vi "PDF Optionen automatisch.vi"(8 "error in (no error)":errorcluster caption="Fehler (Eingang, kein Fehler)", 9 "PDF Optionen Referenzen Cluster":T1, 10 "Anzahl aktive Komponenten":i32, 11 "PDF Optionen (Eingang)":T2) -> (0 "error out":errorcluster caption="Fehler (Ausgang)", 2 "Anzahl aktive Komponenten out":i32, 3 "PDF Optionen (Ausgang)":T2, 4 "PDF Einzelseiten Span":bool, 5 "PDF öffnen":bool, 6 "PDF Einzelseiten Komponenten":bool, 7 "PDF Deckblatt":bool)   [LabVIEW 2020, in "Linearisierung v2.lvlib" / "Protokoll.lvlib"]
uses:
  Protokoll.lvlib
  SpanEinstellungen/PDF Optionen.ctl
  SpanEinstellungen/SpanEinstellungen.lvlib
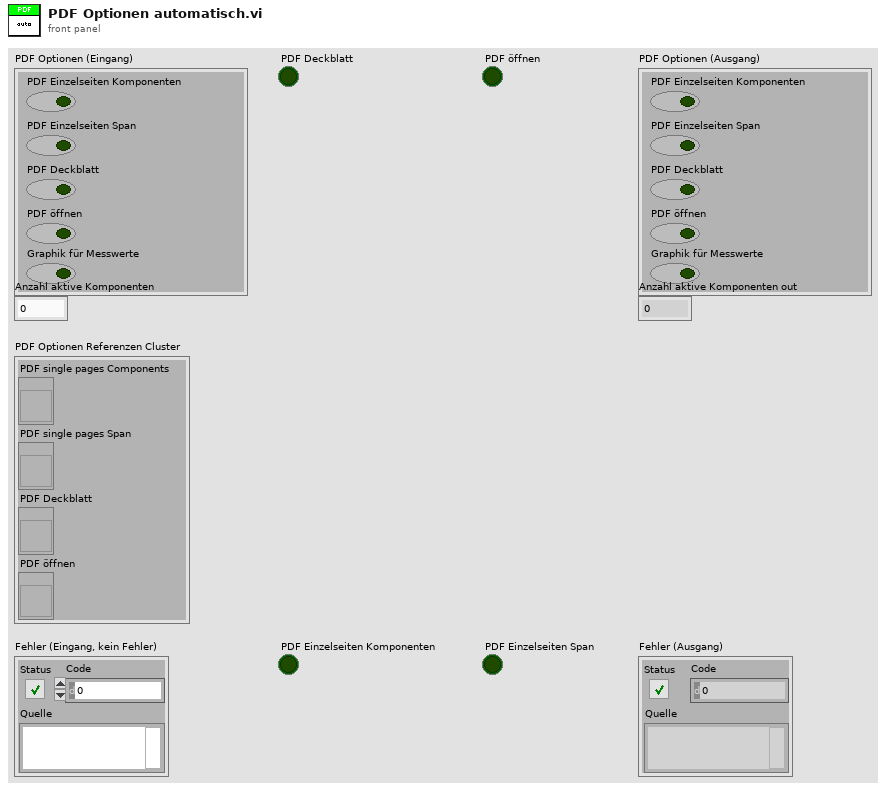
[diagram p1: front panel]
types:
  T1 = cluster{"PDF single pages Components":refnum<vi>, "PDF single pages Span":refnum<vi>, "PDF Deckblatt":refnum<vi>, "PDF öffnen":refnum<vi>}
  T2 = typedef "Linearisierung v2.lvlib/SpanEinstellungen.lvlib/PDF Optionen.ctl" = cluster{"PDF Einzelseiten Komponenten":bool, "PDF Einzelseiten Span":bool, "PDF Deckblatt":bool, "PDF öffnen":bool, "Graphik für Messwerte":bool}
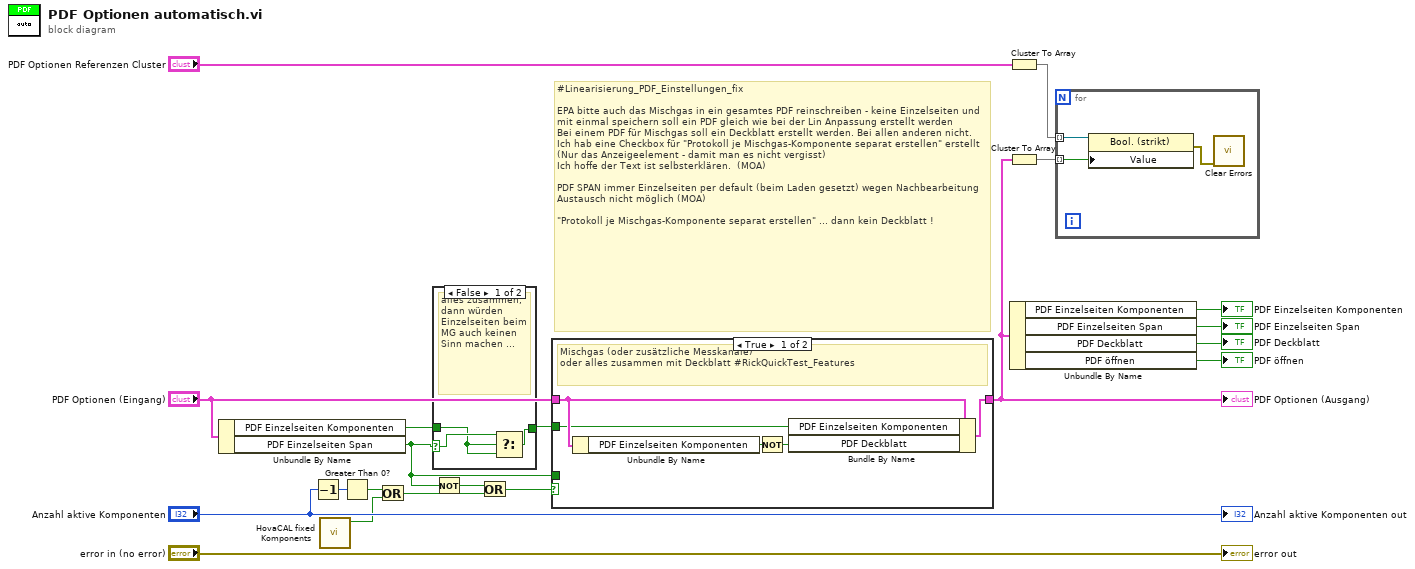
[diagram p0: block diagram]
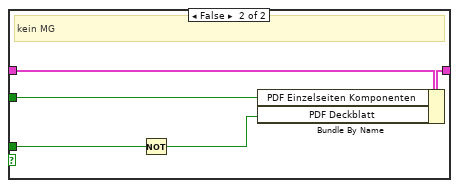
[diagram p3: hidden frame]
diagram:
  # "#Linearisierung_PDF_Einstellungen_fix\n\nEPA bitte auch das Mischgas in ein gesamtes PDF reinschreiben - keine Einzelseiten und mit einmal speichern soll ein PDF gleich wie bei der Lin Anpassung erstellt werden\nBei einem PDF für Mischgas soll ein Deckblatt erstellt werden. Bei allen anderen nicht. \nIch hab eine Checkbox für \"Protokoll je Mischgas-Komponente separat erstellen\" erstellt (Nur das Anzeigeelement - damit man es nicht vergisst)\nIch hoffe der Text ist selbsterklären.  (MOA)\n\nPDF SPAN immer Einzelseiten per default (beim Laden gesetzt) wegen Nachbearbeitung Austausch nicht möglich (MOA) \n\n\"Protokoll je Mischgas-Komponente separat erstellen\" ... dann kein Deckblatt !"
  n1 = Unbundle By Name("PDF Optionen (Eingang)") -> ("PDF Einzelseiten Komponenten"=w10:bool, "PDF Einzelseiten Span"=w4:bool)
  n2 = Decrement(x="Anzahl aktive Komponenten") -> (x-1=w18:i32)
  n3 = call "HovaCAL fixed Komponents.vi"() -> ("HovaCAL fixed"=w1:bool)  [unwired: 10 in, 1 out]
  n4 = Greater Than 0?(x=w18) -> (x > 0?=w19:bool)
  n5 = Or(x=w19, y=w1) -> (x .or. y?=w2:bool)
  n6 = case shown="False" w4 {
    selector: w4 -> [w23 _]
    tunnel: w10 -> [w22 w24]
    tunnel: [w21 w24] -> w9
    frame False {
      # "alles zusammen, dann würden Einzelseiten beim MG auch keinen Sinn machen ..."
      n7 = Select(t=w23, s=w22, f=w22) -> (s? t:f=w21:bool)
    }
    frame True {
      # "Standard alles einezln"
    }
  }
  n8 = Not(x=w4) -> (.not. x?=w3:bool)
  n9 = Or(x=w3, y=w2) -> (x .or. y?=w5:bool)
  n10 = case shown="True" w5 {
    tunnel: "PDF Optionen (Eingang)" -> [w28 w33]
    tunnel: [w29 w34] -> w14
    tunnel: w9 -> [w25 w32]
    tunnel: w4 -> [_ w31]
    frame True {
      # "Mischgas (oder zusätzliche Messkanäle)\noder alles zusammen mit Deckblatt #RickQuickTest_Features"
      n11 = Unbundle By Name(w28) -> ("PDF Einzelseiten Komponenten"=w27:bool)
      n12 = Not(x=w27) -> (.not. x?=w26:bool)
      n13 = Bundle By Name(cluster=w28, "PDF Einzelseiten Komponenten"=w25, "PDF Deckblatt"=w26) -> (w29:T2)
    }
    frame False {
      # "kein MG"
      n14 = Not(x=w31) -> (.not. x?=w30:bool)
      n15 = Bundle By Name(cluster=w33, "PDF Einzelseiten Komponenten"=w32, "PDF Deckblatt"=w30) -> (w34:T2)
    }
  }
  "PDF Optionen (Ausgang)" <- w14
  n16 = Cluster To Array(cluster="PDF Optionen Referenzen Cluster") -> (array=w6:refnum<vi>[])
  n17 = Cluster To Array(cluster=w14) -> (array=w13:bool[])
  n18 = Unbundle By Name(w14) -> ("PDF Einzelseiten Komponenten"=→"PDF Einzelseiten Komponenten":bool, "PDF Einzelseiten Span"=→"PDF Einzelseiten Span":bool, "PDF Deckblatt"=→"PDF Deckblatt":bool, "PDF öffnen"=→"PDF öffnen":bool)
  n19 = for {
    tunnel: w6 -> [w37] mode=indexing
    tunnel: w13 -> [w36] mode=indexing
    n20 = property class="Bool. (strikt)"(reference=w37, "Value"=w36) -> (error out=w35:errorcluster)  [unwired: 1 in, 1 out]
    n21 = call <vilib>:"Clear Errors.vi"("error in (no error)"=w35) -> ()  [unwired: 5 in, 2 out]
  }
  "Anzahl aktive Komponenten out" <- "Anzahl aktive Komponenten"
  "error out" <- "error in (no error)"
